vi "Decision to Report Dose.vi"(9 "Timer Elapsed or Sets # Reached?":bool, 10 "Measurement Information":T1={"Comments"="", "Directory Input"="", "Data file path"=path "C:/Data/EPR Data", "Scripting File"=path "C:/Data/Configuration Script.csv", "Save Data"=FALSE, "Tooth size (d11) [mm]"=0.0, "Tooth size (d12) [mm]"=0.0, "Tooth size (d21) [mm]"=0.0, "Tooth size (d22) [mm]"=0.0, "Dose of Tooth [Gy]"=0.0, "Safe Shutdown?"=FALSE, "Gases Available"=[], "Database Username"="", "Database Password"="", "Database Login URL"="", "Database Upload URL"="", "Database Success URL"="", "Database XML URL"="", "Database Resonator URL"="", "Session Number"=0, "Set #"=0, "Resonator Operator"="", "Session Type"="", "Tooth/Sample ID"="", "Volunteer ID"="", "Computer Operator"="", "Volunteer Type"="", "Site/Tooth Selection (T8,T9)"="", "Resonator"="", "Measurement Site"="", "Non-standard session?"=FALSE, "EPR DAQ Version"="", "Session Path"=path "C:/Data/EPR Data", "Chosen Applied State"="", "Chosen Initial State"="", "Time of Transition"="", "DAQ Mode"=enum."Engineering", "pO2/Scan [mmHg]"=[], "pO2/Set [mmHg]"=[], "Linewidth (HWHM)/Scan [Gauss]"=[], "Linewidth (HWHM)/Set [Gauss]"=[], "pO2 Conversion"="", "Dose Calibration Cluster"={"Dose Response"={"grand_mean"=0.0292016, "slope"=0.0188720543}, "Dose Correction"={"Sex"=1, "a0"=7.719669421, "a1"=-2.746550736, "a2"=-0.186490355, "a3"=0.041922063, "a4"=-0.849147359, "a5"=0.14330063, "a6"=0.019930219, "A_n"=40.0, "H_n"=10.12, "Dose Correction"=FALSE}, "Dose Reporting"={"Reporting is"=TRUE, "sd_threshold [AU]"=0.06, "sd_model [Gy]"=0.66, "dosimetric_threshold [Gy]"=2.0, "Add intrasession errors is"=FALSE, "Prior Radiation?"=FALSE}}, "OxyChip Slope"=0.0, "OxyChip Intercept"=0.0, "QA Mode"=enum."Select QA Mode", "QA Session?"=FALSE, "Sample Type"=enum."Empty Resonator", "Report pO2/Scan"=FALSE, "Skip End Session Save"=FALSE, "Number of sites"=enum."# Probes", "Recipient Name"="", "Sender Name"="", "Recipient Email"="", "Transition State History"=[], "pO2 Report Times"=[], "Temperature [C]"=0.0, "+Error pO2/Scan [mmHg]"=[], "-Error pO2/Scan [mmHg]"=[], "+Error pO2/Set [mmHg]"=[], "-Error pO2/Set [mmHg]"=[], "Oxy Phase Exclusion Tolerance [rad]"=0.0, "Oxy Center Exclusion Tolerance [%]"=0.0, "Oxy Exclude Unacceptable"=FALSE, "Oxy Unacceptable Estimate Flags"=[], "Save Session PPT"=FALSE, "Flagged Bad Sets"=[]} {"Oxy Center Exclusion Tolerance [%]" format="%#_9g"; "Oxy Phase Exclusion Tolerance [rad]" format="%#_9g"; "Temperature [C]" format="%#_9g"; "OxyChip Intercept" format="%#_9g"; "OxyChip Slope" format="%#_9g"; "Dose Calibration Cluster"."Dose Reporting"."dosimetric_threshold [Gy]" format="%#_9g"; "Dose Calibration Cluster"."Dose Reporting"."sd_model [Gy]" format="%#_9g"; "Dose Calibration Cluster"."Dose Reporting"."sd_threshold [AU]" format="%#_9g"; "Dose Calibration Cluster"."Dose Correction"."H_n" format="%#_9g"; "Dose Calibration Cluster"."Dose Correction"."A_n" format="%#_9g"; "Dose Calibration Cluster"."Dose Correction"."a6" format="%#.9g"; "Dose Calibration Cluster"."Dose Correction"."a5" format="%#.9g"; "Dose Calibration Cluster"."Dose Correction"."a4" format="%#.9g"; "Dose Calibration Cluster"."Dose Correction"."a3" format="%#.9g"; "Dose Calibration Cluster"."Dose Correction"."a2" format="%#.9g"; "Dose Calibration Cluster"."Dose Correction"."a1" format="%#.9g"; "Dose Calibration Cluster"."Dose Correction"."a0" format="%#.9g"; "Dose Calibration Cluster"."Dose Correction"."Sex" items=["Male"=1, "Female"=0]; "Dose Calibration Cluster"."Dose Response"."slope" format="%#_9g"; "Dose Calibration Cluster"."Dose Response"."grand_mean" format="%#_9g"}, 11 "Acquisition Parameters":T4={"Magnet Angle [deg]"=0.0, "Magnet Angles [deg]"=[], "DeltaVpp [v]"=0.0, "SEM [v]"=0.0, "DeltaVpp Thresh [v]"=0.0, "SEM Thresh [v]"=0.0, "Adaptive Processing"=FALSE, "Acquire Q"=FALSE, "Acquire Photos"=FALSE, "Adaptive Tuning"=FALSE, "Automated Matching"=FALSE, "X-Gradient [G/mm]"=0.0, "Y-Gradient [G/mm]"=0.0, "Z-Gradient [G/mm]"=0.0, "Central Field [G]"=0.0, "Scan Width [G]"=0.0, "Mod. Amp. [G]"=0.0, "Scan Time [s]"=0.0, "Pre-Scan Delay [ms]"=0, "Measurement Timeout [s]"=0.0, "Electromagnet Main Field [G]"=0.0, "Locked Central Field [G]"=0.0, "Scans Excluded"=0, "Scans Completed"=0, "No. Scans/Set"=0, "No. Scans for SNR"=0, "Field Locked Frequency [GHz]"=0.0, "Auto Set-based Field Center"=FALSE, "Prompt for oxy acquisition updates"=FALSE, "Oxy QA Scan?"=FALSE, "Exclude Bad Data"=FALSE, "Optimizing RF Power"=FALSE, "Gradients on/off"=FALSE, "Running Script"=TRUE, "Opto-Coupler Current [A]"=0.0, "Continuous Sweeping"=FALSE, "Sweep Rise Time [sec]"=0, "Reverse Sweep Central Field [G]"=0.0, "Forward Sweep Central Field [G]"=0.0, "Sweep Calibrated"=FALSE, "Modulation Calibrated"=FALSE, "First CheckCal Scan?"=FALSE, "AFC Field Correction"=FALSE, "OxyQAInit Scan Width [G]"=0.0, "OxyQAInit Mod. Amp. [G]"=0.0, "Scans Completed/Session"=0, "Acquire SpO2"=FALSE, "Acquire Temperature"=FALSE, "Over Mod"=FALSE} {"OxyQAInit Mod. Amp. [G]" min=0.0; "OxyQAInit Scan Width [G]" min=0.0; "Mod. Amp. [G]" min=0.0; "Scan Width [G]" min=0.0; "Measurement Timeout [s]" min=0.0; "Scan Time [s]" min=0.0; "Z-Gradient [G/mm]" min=0.0; "Y-Gradient [G/mm]" min=0.0; "X-Gradient [G/mm]" min=0.0; "SEM Thresh [v]" min=0.0; "DeltaVpp Thresh [v]" min=0.0; "SEM [v]" min=0.0}) -> (0 "Report for Adaptive?":bool, 3 "Report Dose?":bool)   [LabVIEW 2016]
uses:
  Types/Acquisition Parameters.ctl
  Types/Measurement Information.ctl
  Analysis/Dose Calculation and Reporting/Dose Calculation Control.ctl
  Types/Sample Type.ctl
panel:
  # "Session Information"
  # "Oximetric Data and Information"
  # "Email"
  # "Tooth Information"
  # "Database"
  # "Gradients"
  # "Field"
  # "Scans and Sets"
  # "Timing"
  # "Adaptive Dosimetric \nData Processing"
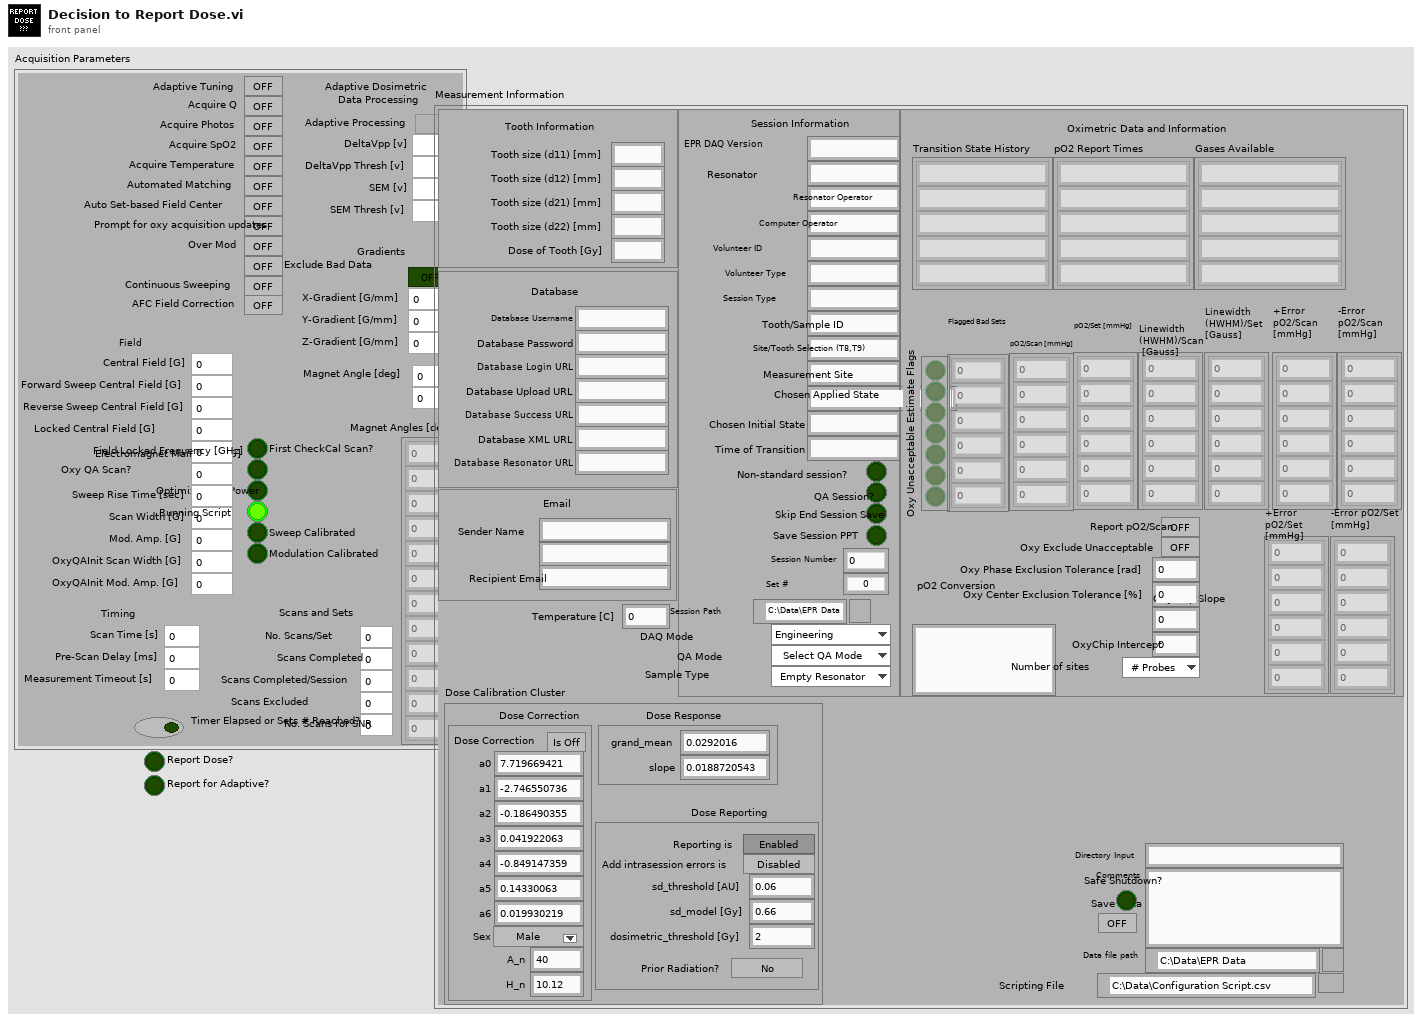
[diagram p1: front panel]
types:
  T1 = typedef "Measurement Information.ctl" = cluster{"Comments":string, "Directory Input":string, "Data file path":path, "Scripting File":path, "Save Data":bool, "Tooth size (d11) [mm]":dbl, "Tooth size (d12) [mm]":dbl, "Tooth size (d21) [mm]":dbl, "Tooth size (d22) [mm]":dbl, "Dose of Tooth [Gy]":dbl, "Safe Shutdown?":bool, "Gases Available":string[], "Database Username":string, "Database Password":string, "Database Login URL":string, "Database Upload URL":string, "Database Success URL":string, "Database XML URL":string, "Database Resonator URL":string, "Session Number":i32, "Set #":u32, "Resonator Operator":string, "Session Type":string, "Tooth/Sample ID":string, "Volunteer ID":string, "Computer Operator":string, "Volunteer Type":string, "Site/Tooth Selection (T8,T9)":string, "Resonator":string, "Measurement Site":string, "Non-standard session?":bool, "EPR DAQ Version":string, "Session Path":path, "Chosen Applied State":string, "Chosen Initial State":string, "Time of Transition":string, "DAQ Mode":enum16{"Engineering", "Dosimetry", "Oximetry"}, "pO2/Scan [mmHg]":dbl[][], "pO2/Set [mmHg]":dbl[][], "Linewidth (HWHM)/Scan [Gauss]":dbl[][], "Linewidth (HWHM)/Set [Gauss]":dbl[][], "pO2 Conversion":string, "Dose Calibration Cluster":T2, "OxyChip Slope":dbl, "OxyChip Intercept":dbl, "QA Mode":enum16{"Select QA Mode", "QA-Start/End", "QA-Mid", "QA-Weekly", "QA-Eng", "Check Calibration"}, "QA Session?":bool, "Sample Type":T3, "Report pO2/Scan":bool, "Skip End Session Save":bool, "Number of sites":enum16{"# Probes", "1", "2", "3", "4"}, "Recipient Name":string, "Sender Name":string, "Recipient Email":string, "Transition State History":string[], "pO2 Report Times":string[], "Temperature [C]":dbl, "+Error pO2/Scan [mmHg]":dbl[][], "-Error pO2/Scan [mmHg]":dbl[][], "+Error pO2/Set [mmHg]":dbl[][], "-Error pO2/Set [mmHg]":dbl[][], "Oxy Phase Exclusion Tolerance [rad]":dbl, "Oxy Center Exclusion Tolerance [%]":dbl, "Oxy Exclude Unacceptable":bool, "Oxy Unacceptable Estimate Flags":bool[], "Save Session PPT":bool, "Flagged Bad Sets":u32[]}
  T2 = typedef "Dose Calculation Control.ctl" = cluster{"Dose Response":cluster{"grand_mean":dbl, "slope":dbl}, "Dose Correction":cluster{"Sex":u16, "a0":dbl, "a1":dbl, "a2":dbl, "a3":dbl, "a4":dbl, "a5":dbl, "a6":dbl, "A_n":dbl, "H_n":dbl, "Dose Correction":bool}, "Dose Reporting":cluster{"Reporting is":bool, "sd_threshold [AU]":dbl, "sd_model [Gy]":dbl, "dosimetric_threshold [Gy]":dbl, "Add intrasession errors is":bool, "Prior Radiation?":bool}}
  T3 = typedef "Sample Type.ctl" = enum16{"Empty Resonator", "IRS", "BallZero", "Irradiated Tooth", "Non-irradiated Tooth", "OxyChip", "LiPc", "PDT", "India Ink"}
  T4 = typedef "Acquisition Parameters.ctl" = cluster{"Magnet Angle [deg]":dbl, "Magnet Angles [deg]":dbl[], "DeltaVpp [v]":dbl, "SEM [v]":dbl, "DeltaVpp Thresh [v]":dbl, "SEM Thresh [v]":dbl, "Adaptive Processing":bool, "Acquire Q":bool, "Acquire Photos":bool, "Adaptive Tuning":bool, "Automated Matching":bool, "X-Gradient [G/mm]":dbl, "Y-Gradient [G/mm]":dbl, "Z-Gradient [G/mm]":dbl, "Central Field [G]":dbl, "Scan Width [G]":dbl, "Mod. Amp. [G]":dbl, "Scan Time [s]":dbl, "Pre-Scan Delay [ms]":u32, "Measurement Timeout [s]":dbl, "Electromagnet Main Field [G]":dbl, "Locked Central Field [G]":dbl, "Scans Excluded":u32, "Scans Completed":u32, "No. Scans/Set":u32, "No. Scans for SNR":u32, "Field Locked Frequency [GHz]":dbl, "Auto Set-based Field Center":bool, "Prompt for oxy acquisition updates":bool, "Oxy QA Scan?":bool, "Exclude Bad Data":bool, "Optimizing RF Power":bool, "Gradients on/off":bool, "Running Script":bool, "Opto-Coupler Current [A]":dbl, "Continuous Sweeping":bool, "Sweep Rise Time [sec]":u32, "Reverse Sweep Central Field [G]":dbl, "Forward Sweep Central Field [G]":dbl, "Sweep Calibrated":bool, "Modulation Calibrated":bool, "First CheckCal Scan?":bool, "AFC Field Correction":bool, "OxyQAInit Scan Width [G]":dbl, "OxyQAInit Mod. Amp. [G]":dbl, "Scans Completed/Session":u32, "Acquire SpO2":bool, "Acquire Temperature":bool, "Over Mod":bool}
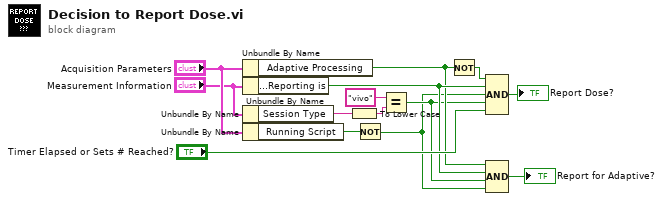
[diagram p0: block diagram]
diagram:
  n1 = Unbundle By Name("Acquisition Parameters") -> ("Adaptive Processing"=w3:bool)
  n2 = Unbundle By Name("Measurement Information") -> ("Dose Calibration Cluster.Dose Reporting.Reporting is"=w4:bool)
  n3 = Unbundle By Name("Measurement Information") -> ("Session Type"=w11:string)
  n4 = Unbundle By Name("Acquisition Parameters") -> ("Running Script"=w10:bool)
  n5 = To Lower Case(string=w11) -> (all lower case string=w12:string)
  n6 = Not(x=w10) -> (.not. x?=w1:bool)
  n7 = Equal?(x="vivo", y=w12) -> (x = y?=w2:bool)
  n8 = Not(x=w3) -> (.not. x?=w14:bool)
  n9 = Compound Arithmetic op=AND(w14, w4, w1, w2, "Timer Elapsed or Sets # Reached?") -> (→"Report Dose?":bool)
  n10 = Compound Arithmetic op=AND(w3, w4, w2, w1) -> (→"Report for Adaptive?":bool)
